vi "stop.vi"(8 "error in (no error)":errorcluster, 11 "FPGAWrapperDL090211Galvo in":refnum<class "FPGAWrapperMM140723Galvo.lvclass">) -> (0 "error out":errorcluster, 3 "FPGAWrapperDL090211Galvo out":refnum<class "FPGAWrapperMM140723Galvo.lvclass">)   [LabVIEW 2010, in "FPGAWrapperMM140723Galvo.lvclass"]
uses:
  FPGAWrapperMM140723Galvo.lvclass
  type definitions/command_enum.ctl
  class_data.vi
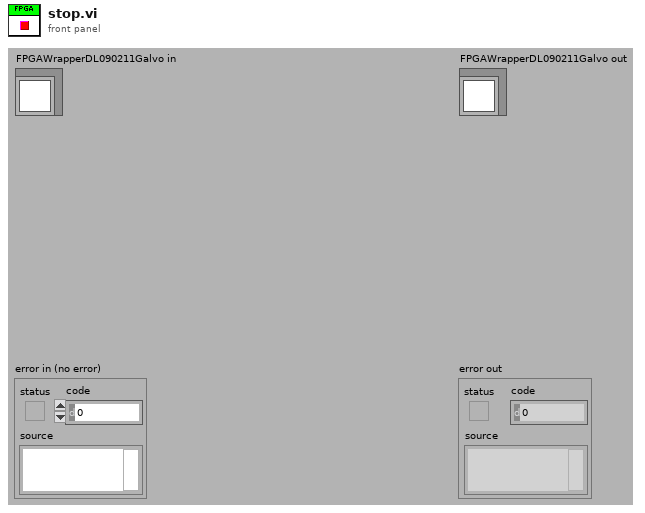
[diagram p1: front panel]
types:
  T1 = typedef "command_enum.ctl" = enum16{"NULL", "update", "start", "stop", "reset", "shut-down"}
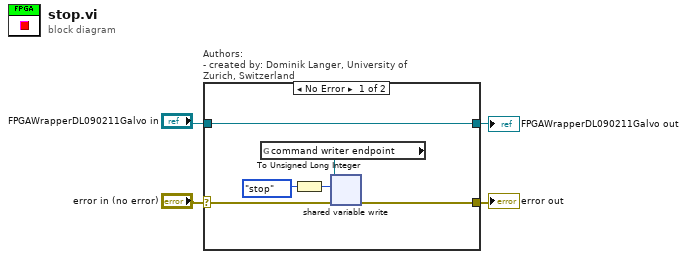
[diagram p0: block diagram]
diagram:
  n1 = case "Authors: \n- created by: Dominik Langer, University of Zurich, Switzerland" shown="No Error" "error in (no error)" {
    selector: "error in (no error)" -> [w7 w11]
    tunnel: "FPGAWrapperDL090211Galvo in" -> [w8 w12]
    tunnel: [w8 w12] -> w2
    tunnel: [w6 w11] -> w3
    frame No Error {
      n2 = global read "class_data.vi" "command writer endpoint"() -> (w5:refnum<k21>)
      n3 = To Unsigned Long Integer(number=command_enum."stop" ("command")) -> (unsigned 32bit integer=w10:u32)
      n4 = shared-variable-write(w5, w7, w10) -> (w6:errorcluster)  [unwired: 1 in, 2 out]
    }
    frame Error {
    }
  }
  "error out" <- w3
  "FPGAWrapperDL090211Galvo out" <- w2
